vi "Reset Supply.vi"(8 "error in":errorcluster, 11 "6032A in":refnum<class "6032A.lvclass">) -> (0 "error out":errorcluster, 3 "6032A out":refnum<class "6032A.lvclass">)   [LabVIEW 2019, in "6032A.lvlib" / "6032A.lvclass"]
uses:
  Library/6032A.lvclass
  Library/6032A.lvclass/6032A.ctl
  builds/Instruments/PowerSupply.lvlibp/Library/PowerSupply.lvclass
  <instrlib>/Agilent 6XXX Series/Agilent 6XXX Series.lvlib
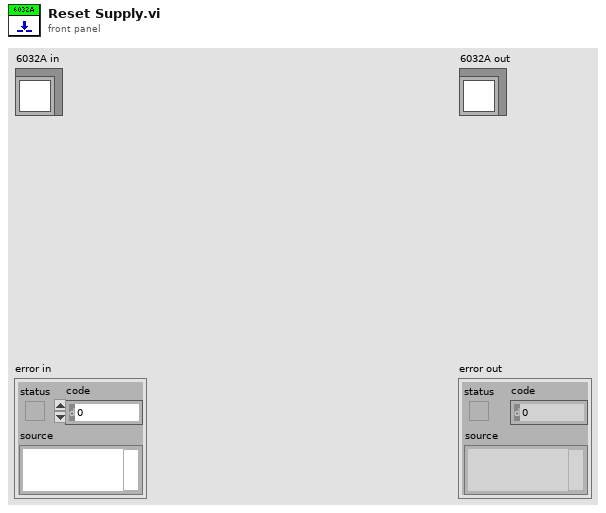
[diagram p1: front panel]
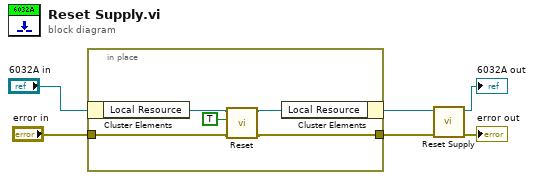
[diagram p0: block diagram]
diagram:
  n1 = in-place {
    in-place-border: "error in" -> [w10]
    in-place-border: [w8] -> w2
    n2 = in-place-cluster #1("6032A in") -> ("Local Resource"=w11:refnum<visa-resource-name>)
    n3 = call <instrlib>:"Reset.vi"("error in (no error)"=w10, "reset (T:device)"=TRUE, "VISA resource name"=w11) -> ("error out"=w8:errorcluster, "VISA resource name out"=w9:refnum<visa-resource-name>)  [unwired: 7 in]
    n4 = in-place-cluster #1("Local Resource"=w9) -> (w1:refnum<class "6032A.lvclass">)
  }
  n5 = call-parent "Reset Supply.vi"("error in"=w2, "PowerSupply in"=w1) -> ("error out"=→"error out":errorcluster, "PowerSupply out"=→"6032A out":refnum<class "6032A.lvclass">)  [unwired: 8 in]
